vi "Dac_Output_cam_trig_multiple_digital_signals_test.vi"(0 "File to read":path=path "C:/Users/lpk27/Documents/pan-ASLMsynched/pan-ASLM/Calibration files/newcalibration_voice coil input_25msflyback.txt", 1 "Image acquisition time (ms)":dbl=1000.0, 2 "Delay between frames":dbl=25.0, 3 "typedef_laser_order_control":T1={"Laser 560 nm order selection"=0, "Laser 595 nm order selection"=0, "Laser 642 nm order selection"=0, "Laser 488 nm order selection"=1, "Color Box"=60927, "Color Box 2"=12844800, "Color Box 3"=14132992, "Color Box 4"=16715008} {"Laser 488 nm order selection" items=["Not active", "1", "2", "3", "4"]; "Laser 642 nm order selection" items=["Not active", "1", "2", "3", "4"]; "Laser 595 nm order selection" items=["Not active", "1", "2", "3", "4"]; "Laser 560 nm order selection" items=["Not active", "1", "2", "3", "4"]}, 4 "stop":bool, 5 "error in":errorcluster, 6 "Number of slices":i32=1000, 11 "Setup":enum16{"Test setup", "Microscope"}(ring)) -> (19 "error out":errorcluster)   [LabVIEW 2020]
uses:
  typedefs/typedef_laser_order_control.ctl
  <vilib>/DAQmx/write.llb/DAQmx Write (Digital Wfm 1Chan NSamp).vi
  <vilib>/DAQmx/write.llb/DAQmx Write (Analog Wfm 1Chan NSamp).vi
  <vilib>/Utility/file.llb/Read Delimited Spreadsheet (DBL).vi
  <vilib>/DAQmx/create/channels.llb/DAQmx Create Channel (AO-Voltage-Basic).vi
  <vilib>/DAQmx/configure/timing.llb/DAQmx Timing (Sample Clock).vi
  <vilib>/DAQmx/miscellaneous.llb/DAQmx Fill In Error Info.vi
  Global stop DAQ.vi
  <vilib>/DAQmx/create/channels.llb/DAQmx Create Channel (CO-Pulse Generation-Ticks).vi
  <vilib>/DAQmx/configure/timing.llb/DAQmx Timing (Implicit).vi
  <vilib>/DAQmx/create/channels.llb/DAQmx Create Channel (DO-Digital Output).vi
  <vilib>/Waveform/DWDTOps.llb/DWDT Uncompress Digital.vi
  <vilib>/DAQmx/create/channels.llb/DAQmx Create Channel (CO-Pulse Generation-Frequency).vi
  Global DAQ started.vi
  Global Counter count.vi
  <resource>/objmgr/daqmx.rc
panel:
  out "CO.Count":u32
  in  "Camera trigger initial delay [s]":dbl format="%.6f"
  out "error out 4":errorcluster
  out "error out 3":errorcluster
  out "error out 2":errorcluster
  out "Digital Waveform Graph":digitalwaveform(graph)
  out "LabVIEW generated Sawtooth input (blue) and Camera trigger (red)":waveform(dbl)(graph)={"t0"=timestamp(0 s since 1904-01-01), "dt"=1.0, "Y"=array[3075 elements]}
  out "# Samples written per channel":u32=3075
  out "actual frequency":dbl=1000.0
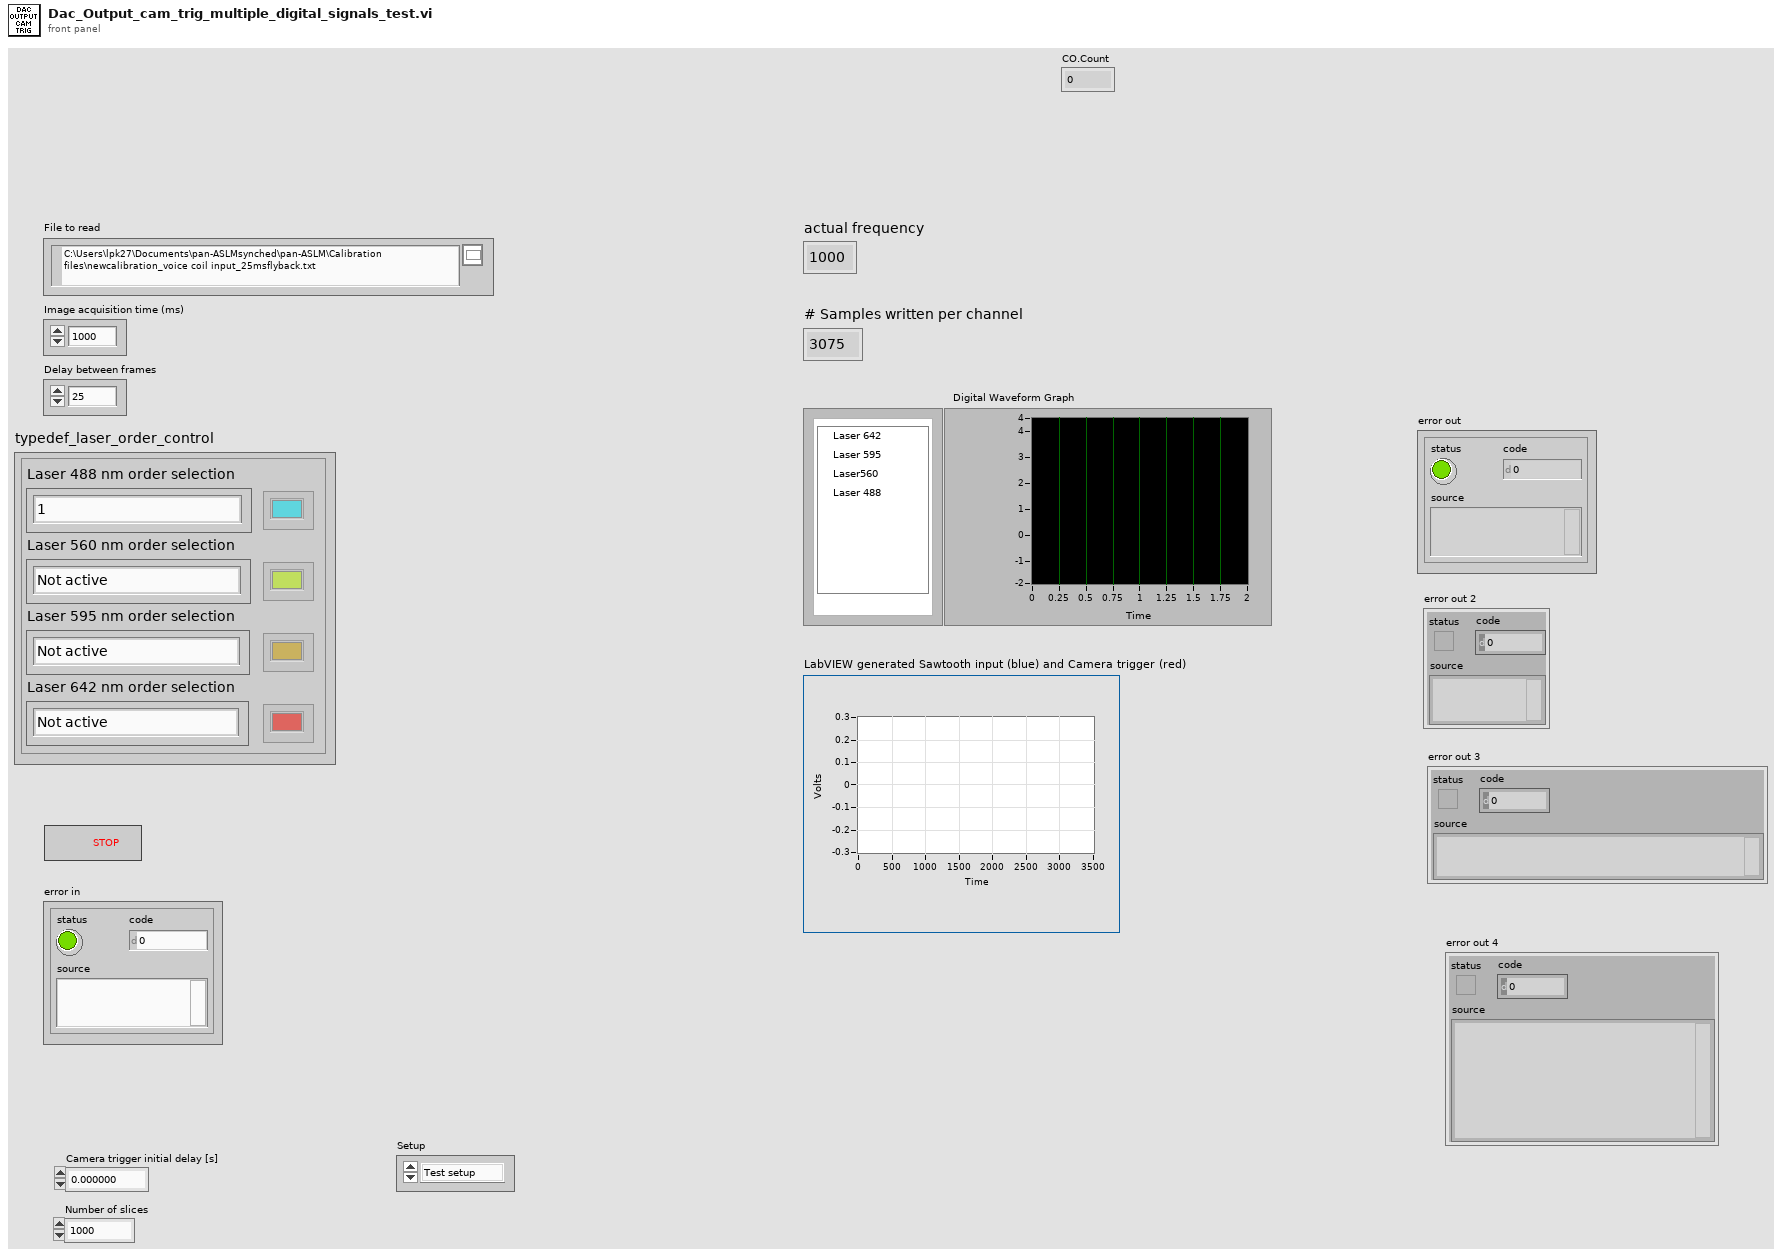
[diagram p1: front panel]
types:
  T1 = typedef "typedef_laser_order_control.ctl" = cluster{"Laser 560 nm order selection":u16, "Laser 595 nm order selection":u16, "Laser 642 nm order selection":u16, "Laser 488 nm order selection":u16, "Color Box":u32, "Color Box 2":u32, "Color Box 3":u32, "Color Box 4":u32}
  T2 = typedef "DAQ_channel_typedef.ctl" = cluster{"CO.Pulse.Term":tag, "Voice coil analog output":tag, "counter":tag, "CO.Pulse.Term 2":tag, "AOTF lines":tag, "counter 2":tag, "CO.Pulse.Term 3":tag, "counter 3":tag}
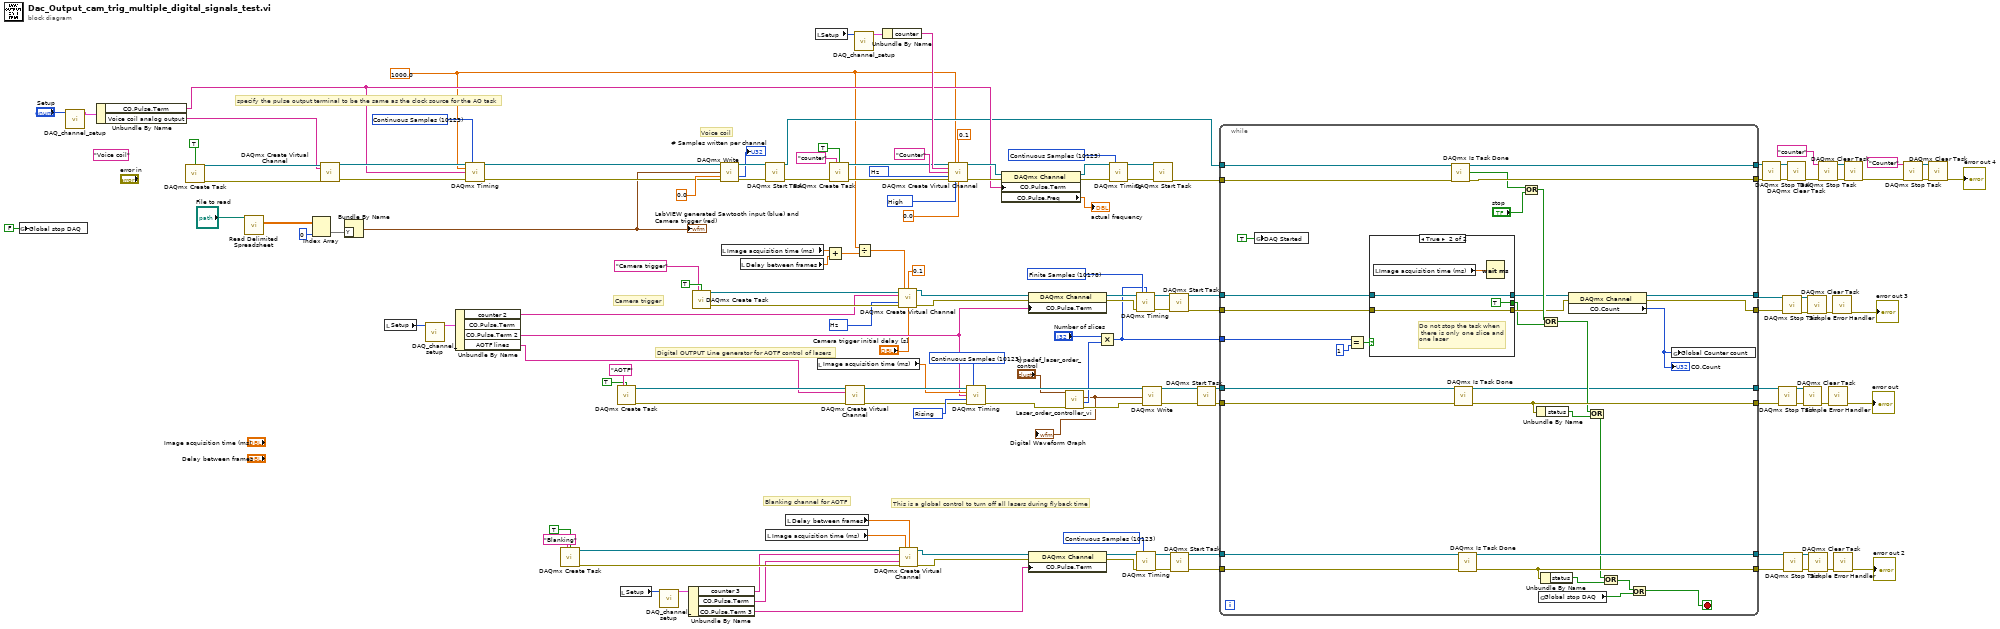
[diagram p0: block diagram]
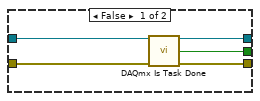
[diagram p2: hidden frame]
diagram:
  w10 = 10373 items=["Hz"=10373] ("units")
  (unwired) "Voice coil" ("new task name")
  w93 = 10123 items=["Finite Samples"=10178, "Continuous Samples"=10123, "Hardware Timed Single Point"=12522] ("sample mode")
  w98 = 10123 items=["Finite Samples"=10178, "Continuous Samples"=10123, "Hardware Timed Single Point"=12522] ("sample mode")
  w106 = 10280 items=["Rising"=10280, "Falling"=10171] ("active edge")
  w116 = 10178 items=["Finite Samples"=10178, "Continuous Samples"=10123, "Hardware Timed Single Point"=12522] ("sample mode")
  w127 = 10192 items=["High"=10192, "Low"=10214] ("idle state")
  w128 = 10373 items=["Hz"=10373] ("units")
  w121 = 10123 items=["Finite Samples"=10178, "Continuous Samples"=10123, "Hardware Timed Single Point"=12522] ("sample mode")
  w9 = 1000.0 ("rate")
  w141 = 10123 items=["Finite Samples"=10178, "Continuous Samples"=10123, "Hardware Timed Single Point"=12522] ("sample mode")
  # "This is a global control to turn off all lasers during flyback time"
  # "Voice coil"
  # "Camera trigger"
  # "Digital OUTPUT Line generator for AOTF control of lasers"
  # "Blanking channel for AOTF"
  # "specify the pulse output terminal to be the same as the clock source for the AO task"
  n1 = global write "Global stop DAQ.vi" "Global stop DAQ"(FALSE ("Global stop DAQ")) -> ()
  n2 = call "DAQ_channel_setup.vi"("Text Ring"="Setup") -> ("DAQ channels OUT"=w38:T2)  [unwired: 10 in]
  n3 = Unbundle By Name(w38) -> ("CO.Pulse.Term"=w17:tag, "Voice coil analog output"=w39:tag)
  n4 = call <vilib>:"DAQmx Create Task.vi"("auto cleanup"=TRUE) -> ("task out"=w75:refnum<k21>, "error out"=w74:errorcluster)  [unwired: 13 in]
  n5 = call-poly <vilib>:"Read Delimited Spreadsheet.vi"("file path (dialog if empty)"="File to read") -> ("all rows"=w112:dbl[][])  [unwired: 9 in, 5 out]
  n6 = Index Array(array=w112, index (col)=0 ("disabled index (col)")) -> (element=w110:dbl[])  [unwired: 1 in]
  n7 = call-poly <vilib>:"DAQmx Create Virtual Channel.vi"("task in"=w75, "physical channels"=w39, "error in"=w74) -> ("task out"=w143:refnum<k21>, "error out"=w142:errorcluster)  [unwired: 11 in]
  n8 = Bundle By Name("Y"=w110) -> (w109:waveform(dbl))  [unwired: 1 in]
  "LabVIEW generated Sawtooth input (blue) and Camera trigger (red)" <- w109
  n9 = local read "Setup"() -> (w27:enum16{"Test setup", "Microscope"})
  n10 = call "DAQ_channel_setup.vi"("Text Ring"=w27) -> ("DAQ channels OUT"=w35:T2)  [unwired: 10 in]
  n11 = Unbundle By Name(w35) -> ("counter 2"=w30:tag, "CO.Pulse.Term 2"=w14:tag, "AOTF lines"=w34:tag)  [unwired: 1 out]
  n12 = call-poly <vilib>:"DAQmx Timing.vi"("task/channels in"=w143, "sample mode"=w141, "rate"=w9, "source"=w17, "error in"=w142) -> ("task out"=w123:refnum<k21>, "error out"=w122:errorcluster)  [unwired: 9 in]
  n13 = call <vilib>:"DAQmx Create Task.vi"("new task name"="Blanking", "auto cleanup"=TRUE) -> ("task out"=w80:refnum<k21>, "error out"=w79:errorcluster)  [unwired: 12 in]
  n14 = call <vilib>:"DAQmx Create Task.vi"("new task name"="AOTF", "auto cleanup"=TRUE) -> ("task out"=w77:refnum<k21>, "error out"=w76:errorcluster)  [unwired: 12 in]
  n15 = local read "Setup"() -> (w28:enum16{"Test setup", "Microscope"})
  n16 = call "DAQ_channel_setup.vi"("Text Ring"=w28) -> ("DAQ channels OUT"=w33:T2)  [unwired: 10 in]
  n17 = Unbundle By Name(w33) -> ("counter 3"=w32:tag, "CO.Pulse.Term"=w21:tag, "CO.Pulse.Term 3"=w31:tag)
  n18 = call <vilib>:"DAQmx Create Task.vi"("new task name"="Camera trigger", "auto cleanup"=TRUE) -> ("task out"=w72:refnum<k21>, "error out"=w73:errorcluster)  [unwired: 12 in]
  n19 = call-poly <vilib>:"DAQmx Write.vi"("task/channels in"=w123, "data"=w109, "timeout"=0.0, "error in"=w122) -> ("task out"=w132:refnum<k21>, "number of samples written per channel"=→"# Samples written per channel":u32, "error out"=w131:errorcluster)  [unwired: 9 in]
  n20 = local read "Image acquisition time (ms)"() -> (w83:dbl)
  n21 = local read "Delay between frames"() -> (w82:dbl)
  n22 = call <vilib>:"DAQmx Start Task.vi"("task/channels in"=w132, "error in"=w131) -> ("task out"=w16:refnum<k21>, "error out"=w126:errorcluster)  [unwired: 12 in]
  n23 = local read "Image acquisition time (ms)"() -> (w85:dbl)
  n24 = local read "Delay between frames"() -> (w84:dbl)
  n25 = local read "Setup"() -> (w26:enum16{"Test setup", "Microscope"})
  n26 = local read "Image acquisition time (ms)"() -> (w88:dbl)
  n27 = Add(x=w83, y=w82) -> (x+y=w13:dbl)
  n28 = call <vilib>:"DAQmx Create Task.vi"("new task name"="counter", "auto cleanup"=TRUE, "error in"=w126) -> ("task out"=w23:refnum<k21>, "error out"=w138:errorcluster)  [unwired: 11 in]
  n29 = call-poly <vilib>:"DAQmx Create Virtual Channel.vi"("task in"=w77, "lines"=w34, "error in"=w76) -> ("task out"=w105:refnum<k21>, "error out"=w104:errorcluster)  [unwired: 11 in]
  n30 = call "DAQ_channel_setup.vi"("Text Ring"=w26) -> ("DAQ channels OUT"=w37:T2)  [unwired: 10 in]
  n31 = Divide(x=w9, y=w13) -> (x/y=w12:dbl)
  n32 = Unbundle By Name(w37) -> ("counter"=w36:tag)
  n33 = call-poly <vilib>:"DAQmx Create Virtual Channel.vi"("task in"=w72, "frequency"=w12, "duty cycle"=0.1, "counter"=w30, "units"=w10, "error in"=w73, "initial delay"="Camera trigger initial delay [s]") -> ("task out"=w120:refnum<k21>, "error out"=w108:errorcluster)  [unwired: 7 in]
  n34 = call-poly <vilib>:"DAQmx Create Virtual Channel.vi"("task in"=w80, "high ticks"=w85, "low ticks"=w84, "counter"=w32, "source of ticks"=w21, "error in"=w79) -> ("task out"=w97:refnum<k21>, "error out"=w90:errorcluster)  [unwired: 8 in]
  n35 = call-poly <vilib>:"DAQmx Create Virtual Channel.vi"("task in"=w23, "frequency"=w9, "duty cycle"=0.1, "counter"=w36, "name to assign"="Counter", "units"=w128, "error in"=w138, "idle state"=w127, "initial delay"=0.0) -> ("task out"=w137:refnum<k21>, "error out"=w136:errorcluster)  [unwired: 5 in]
  n36 = call-poly <vilib>:"DAQmx Timing.vi"("task/channels in"=w105, "sample mode"=w98, "rate"=w88, "source"=w14, "active edge"=w106, "error in"=w104) -> ("task out"=w101:refnum<k21>, "error out"=w87:errorcluster)  [unwired: 8 in]
  n37 = property class="DAQmx Channel"(reference=w137, error in=w136, "CO.Pulse.Term"=w17) -> (reference out=w134:refnum<k21>, error out=w135:errorcluster, "CO.Pulse.Freq"=→"actual frequency":dbl)
  n38 = property class="DAQmx Channel"(reference=w120, error in=w108, "CO.Pulse.Term"=w14) -> (reference out=w107:refnum<k21>, error out=w117:errorcluster)
  n39 = property class="DAQmx Channel"(reference=w97, error in=w90, "CO.Pulse.Term"=w31) -> (reference out=w89:refnum<k21>, error out=w94:errorcluster)
  n40 = call "Laser_order_controller_vi.vi"("error in"=w87, "typedef_laser_order_control"="typedef_laser_order_control") -> ("error out"=w86:errorcluster, "Active lasers"=w4:i16, "Digital Waveform Graph"=w3:digitalwaveform)  [unwired: 7 in]
  "Digital Waveform Graph" <- w3
  n41 = Multiply(x="Number of slices", y=w4) -> (x*y=w2:i32)
  n42 = call-poly <vilib>:"DAQmx Timing.vi"("task/channels in"=w134, "sample mode"=w121, "error in"=w135) -> ("task out"=w140:refnum<k21>, "error out"=w139:errorcluster)  [unwired: 11 in]
  n43 = call-poly <vilib>:"DAQmx Timing.vi"("task/channels in"=w107, "sample mode"=w116, "samples per channel"=w2, "error in"=w117) -> ("task out"=w115:refnum<k21>, "error out"=w114:errorcluster)  [unwired: 10 in]
  n44 = call-poly <vilib>:"DAQmx Timing.vi"("task/channels in"=w89, "sample mode"=w93, "error in"=w94) -> ("task out"=w92:refnum<k21>, "error out"=w91:errorcluster)  [unwired: 11 in]
  n45 = call-poly <vilib>:"DAQmx Write.vi"("task/channels in"=w101, "data"=w3, "error in"=w86) -> ("task out"=w103:refnum<k21>, "error out"=w102:errorcluster)  [unwired: 10 in, 1 out]
  n46 = call <vilib>:"DAQmx Start Task.vi"("task/channels in"=w140, "error in"=w139) -> ("error out"=w133:errorcluster)  [unwired: 12 in, 1 out]
  n47 = call <vilib>:"DAQmx Start Task.vi"("task/channels in"=w115, "error in"=w114) -> ("task out"=w119:refnum<k21>, "error out"=w118:errorcluster)  [unwired: 12 in]
  n48 = call <vilib>:"DAQmx Start Task.vi"("task/channels in"=w92, "error in"=w91) -> ("task out"=w96:refnum<k21>, "error out"=w95:errorcluster)  [unwired: 12 in]
  n49 = call <vilib>:"DAQmx Start Task.vi"("task/channels in"=w103, "error in"=w102) -> ("task out"=w100:refnum<k21>, "error out"=w99:errorcluster)  [unwired: 12 in]
  n50 = while {
    tunnel: w133 -> [w177]
    tunnel: w16 -> [w176]
    tunnel: w119 -> [w175]
    tunnel: w118 -> [w174]
    tunnel: w100 -> [w173]
    tunnel: w99 -> [w172]
    tunnel: w96 -> [w171]
    tunnel: w95 -> [w170]
    tunnel: [w169] -> w57
    tunnel: [w163] -> w56
    tunnel: [w153] -> w62
    tunnel: [w151] -> w61
    tunnel: [w155] -> w51
    tunnel: [w168] -> w50
    tunnel: [w167] -> w49
    tunnel: [w166] -> w48
    tunnel: w2 -> [w147]
    stop <- w148 stop-if-true
    n51 = global write "Global DAQ started.vi" "DAQ Started"(TRUE ("DAQ Started")) -> ()
    n52 = Equal?(x=w147, y=1) -> (x = y?=w145:bool)
    n53 = case shown="True" w145 {
      tunnel: w175 -> [w182 w186]
      tunnel: w174 -> [w181 w185]
      tunnel: [w180 w186] -> w154
      tunnel: [w179 w185] -> w152
      tunnel: [w178 TRUE ("task done?")] -> w149
      frame False {
        n54 = call <vilib>:"DAQmx Is Task Done.vi"("task/channels in"=w182, "error in"=w181) -> ("task out"=w180:refnum<k21>, "task done?"=w178:bool, "error out"=w179:errorcluster)  [unwired: 11 in]
      }
      frame True {
        # "Do not stop the task when\n there is only one slice and \none laser"
        n55 = local read "Image acquisition time (ms)"() -> (w183:dbl)
        n56 = Wait (ms)(milliseconds to wait=w183) -> ()  [unwired: 1 out]
      }
    }
    n57 = call <vilib>:"DAQmx Is Task Done.vi"("task/channels in"=w176, "error in"=w177) -> ("task out"=w169:refnum<k21>, "task done?"=w144:bool, "error out"=w163:errorcluster)  [unwired: 11 in]
    n58 = call <vilib>:"DAQmx Is Task Done.vi"("task/channels in"=w173, "error in"=w172) -> ("task out"=w155:refnum<k21>, "error out"=w168:errorcluster)  [unwired: 11 in, 1 out]
    n59 = call <vilib>:"DAQmx Is Task Done.vi"("task/channels in"=w171, "error in"=w170) -> ("task out"=w167:refnum<k21>, "error out"=w166:errorcluster)  [unwired: 11 in, 1 out]
    n60 = Or(x=w144, y="stop") -> (x .or. y?=w157:bool)
    n61 = Unbundle By Name(w168) -> ("status"=w162:bool)
    n62 = global read "Global stop DAQ.vi" "Global stop DAQ"() -> (w159:bool)
    n63 = Unbundle By Name(w166) -> ("status"=w160:bool)
    n64 = Or(x=w157, y=w149) -> (x .or. y?=w165:bool)
    n65 = property class="DAQmx Channel"(reference=w154, error in=w152) -> (reference out=w153:refnum<k21>, error out=w151:errorcluster, "CO.Count"=w150:u32)
    "CO.Count" <- w150
    n66 = Or(x=w165, y=w162) -> (x .or. y?=w164:bool)
    n67 = Or(x=w164, y=w160) -> (x .or. y?=w161:bool)
    n68 = Or(x=w161, y=w159) -> (x .or. y?=w148:bool)
    n69 = global write "Global Counter count.vi" "Global Counter count"(w150) -> ()
  }
  n70 = call <vilib>:"DAQmx Stop Task.vi"("task/channels in"=w57, "error in"=w56) -> ("task out"=w60:refnum<k21>, "error out"=w59:errorcluster)  [unwired: 12 in]
  n71 = call <vilib>:"DAQmx Stop Task.vi"("task/channels in"=w51, "error in"=w50) -> ("task out"=w54:refnum<k21>, "error out"=w55:errorcluster)  [unwired: 12 in]
  n72 = call <vilib>:"DAQmx Stop Task.vi"("task/channels in"=w62, "error in"=w61) -> ("task out"=w65:refnum<k21>, "error out"=w66:errorcluster)  [unwired: 12 in]
  n73 = call <vilib>:"DAQmx Stop Task.vi"("task/channels in"=w49, "error in"=w48) -> ("task out"=w46:refnum<k21>, "error out"=w47:errorcluster)  [unwired: 12 in]
  n74 = call <vilib>:"DAQmx Clear Task.vi"("task in"=w60, "error in"=w59) -> ("error out"=w41:errorcluster)  [unwired: 13 in]
  n75 = call <vilib>:"DAQmx Clear Task.vi"("task in"=w54, "error in"=w55) -> ("error out"=w53:errorcluster)  [unwired: 13 in]
  n76 = call <vilib>:"DAQmx Clear Task.vi"("task in"=w65, "error in"=w66) -> ("error out"=w64:errorcluster)  [unwired: 13 in]
  n77 = call <vilib>:"DAQmx Clear Task.vi"("task in"=w46, "error in"=w47) -> ("error out"=w45:errorcluster)  [unwired: 13 in]
  n78 = call <vilib>:"DAQmx Stop Task.vi"("task/channels in"="counter" ("new task name"), "error in"=w41) -> ("task out"=w43:refnum<k21>, "error out"=w42:errorcluster)  [unwired: 12 in]
  n79 = call <vilib>:"Simple Error Handler.vi"("error in (no error)"=w53) -> ("error out"=→"error out":errorcluster)  [unwired: 4 in, 4 out]
  n80 = call <vilib>:"Simple Error Handler.vi"("error in (no error)"=w64) -> ("error out"=→"error out 3":errorcluster)  [unwired: 4 in, 4 out]
  n81 = call <vilib>:"Simple Error Handler.vi"("error in (no error)"=w45) -> ("error out"=→"error out 2":errorcluster)  [unwired: 4 in, 4 out]
  n82 = call <vilib>:"DAQmx Clear Task.vi"("task in"=w43, "error in"=w42) -> ("error out"=w40:errorcluster)  [unwired: 13 in]
  n83 = call <vilib>:"DAQmx Stop Task.vi"("task/channels in"="Counter" ("new task name"), "error in"=w40) -> ("task out"=w19:refnum<k21>, "error out"=w20:errorcluster)  [unwired: 12 in]
  n84 = call <vilib>:"DAQmx Clear Task.vi"("task in"=w19, "error in"=w20) -> ("error out"=→"error out 4":errorcluster)  [unwired: 13 in]
